vi "CMD_AEROSCRIPTSTATUS.vi"(6 "Gantry in":refnum<class "Gantry.lvclass">, 8 "error in (no error)":errorcluster, 10 "Arguments":string[](array[string]), 11 "gScript Interpreter in":refnum<class "gScript Interpreter.lvclass">) -> (0 "error out":errorcluster, 3 "gScript Interpreter out":refnum<class "gScript Interpreter.lvclass">, 4 "Gantry out":refnum<class "Gantry.lvclass">)   [LabVIEW 2023, in "gScript Interpreter.lvclass"]
uses:
  gScript Interpreter.lvclass
  Shared Components/Gantry Class/Gantry.lvclass
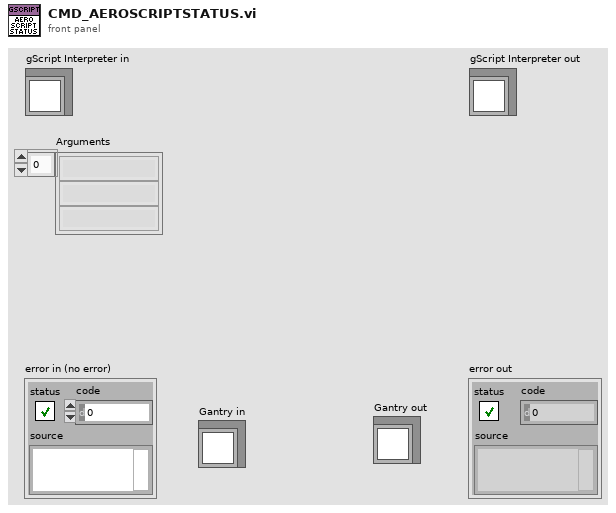
[diagram p1: front panel]
types:
  T1 = enum16{"TLibrary", "T01", "T02", "T03", "T04", "T05", "T06", "T07", "T08", "T09", "T10", "T11", "T12", "T13", "T14", "T15", "T16", "T17", "T18", "T19", "T20", "T21", "T22", "T23", "T24", "T25", "T26", "T27", "T28", "T29", "T30", "T31"}
  T2 = typedef "Memory Cell.ctl" = cluster{"type":T3, "x":dbl, "y":dbl, "z":dbl, "w":dbl}
  T3 = typedef "Memory Cell Type Enum.ctl" = enum16{"integer", "float", "vector", "rotation"}
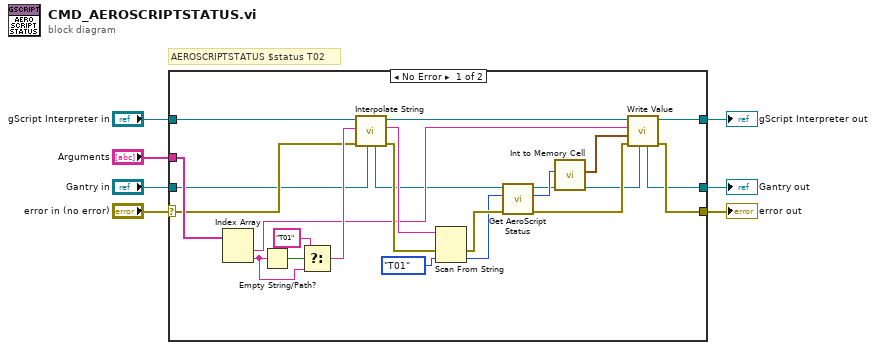
[diagram p0: block diagram]
diagram:
  # "AEROSCRIPTSTATUS $status T02"
  n1 = case shown="No Error" "error in (no error)" {
    selector: "error in (no error)" -> [w22 w33]
    tunnel: [w17 w33] -> w6
    tunnel: [w16 w32] -> w4
    tunnel: "gScript Interpreter in" -> [w23 w32]
    tunnel: "Arguments" -> [w30 _]
    tunnel: "Gantry in" -> [w11 w31]
    tunnel: [w8 w31] -> w1
    frame No Error {
      n2 = Index Array(array=w30) -> (element #1=w18:string, element #2=w21:string)  [unwired: 2 in]
      n3 = Empty String/Path?(string/path=w21) -> (empty?=w27:bool)
      n4 = Select(t="T01", s=w27, f=w21) -> (s? t:f=w25:string)
      n5 = call-dynamic "Interpolate String.vi"("Gantry in"=w11, "error in (no error)"=w22, "Input String"=w25, "gScript Interpreter in"=w23) -> ("error out"=w24:errorcluster, "Output String"=w28:string, "gScript Interpreter out"=w20:refnum<class "gScript Interpreter.lvclass">, "Gantry out"=w10:refnum<class "Gantry.lvclass">)  [unwired: 4 in]
      n6 = Scan From String(input string=w28, error in=w24, default 1=T1."T01" ("taskId")) -> (error out=w15:errorcluster, output 1=w14:T1)  [unwired: 2 in, 2 out]
      n7 = call "Get AeroScript Status.vi"("error in (no error)"=w15, "taskId"=w14, "Gantry in"=w10) -> ("error out"=w13:errorcluster, "State"=w12:i32, "Gantry out"=w9:refnum<class "Gantry.lvclass">)  [unwired: 6 in]
      n8 = call "Int to Memory Cell.vi"("Numeric"=w12) -> ("Memory Cell"=w19:T2)  [unwired: 10 in]
      n9 = call-dynamic "Write Value.vi"("Gantry in"=w9, "error in (no error)"=w13, "Value"=w19, "Address"=w18, "gScript Interpreter in"=w20) -> ("error out"=w17:errorcluster, "gScript Interpreter out"=w16:refnum<class "gScript Interpreter.lvclass">, "Gantry out"=w8:refnum<class "Gantry.lvclass">)  [unwired: 4 in]
    }
    frame Error {
    }
  }
  "error out" <- w6
  "gScript Interpreter out" <- w4
  "Gantry out" <- w1
